vi "PLAN IN UNLOADING SCREEN.vi"(11 "Unloading cyc Data":T1) -> (0 "Unloading cyc Data 2":T1, 1 "Bin/Box":i32, 2 "PLAN DATA Out":string[][](array[string]), 3 "CURRENT PLAN":T2, 5 "FEED CMPLT?":bool)   [LabVIEW 2017]
uses:
  Controls/Unloading_Cyc_Data.ctl
panel:
  # "DOOR NUMBER"
  # "FEEDER STATUS"
  # "DOOR NUMBER"
  # "FEEDER STATUS"
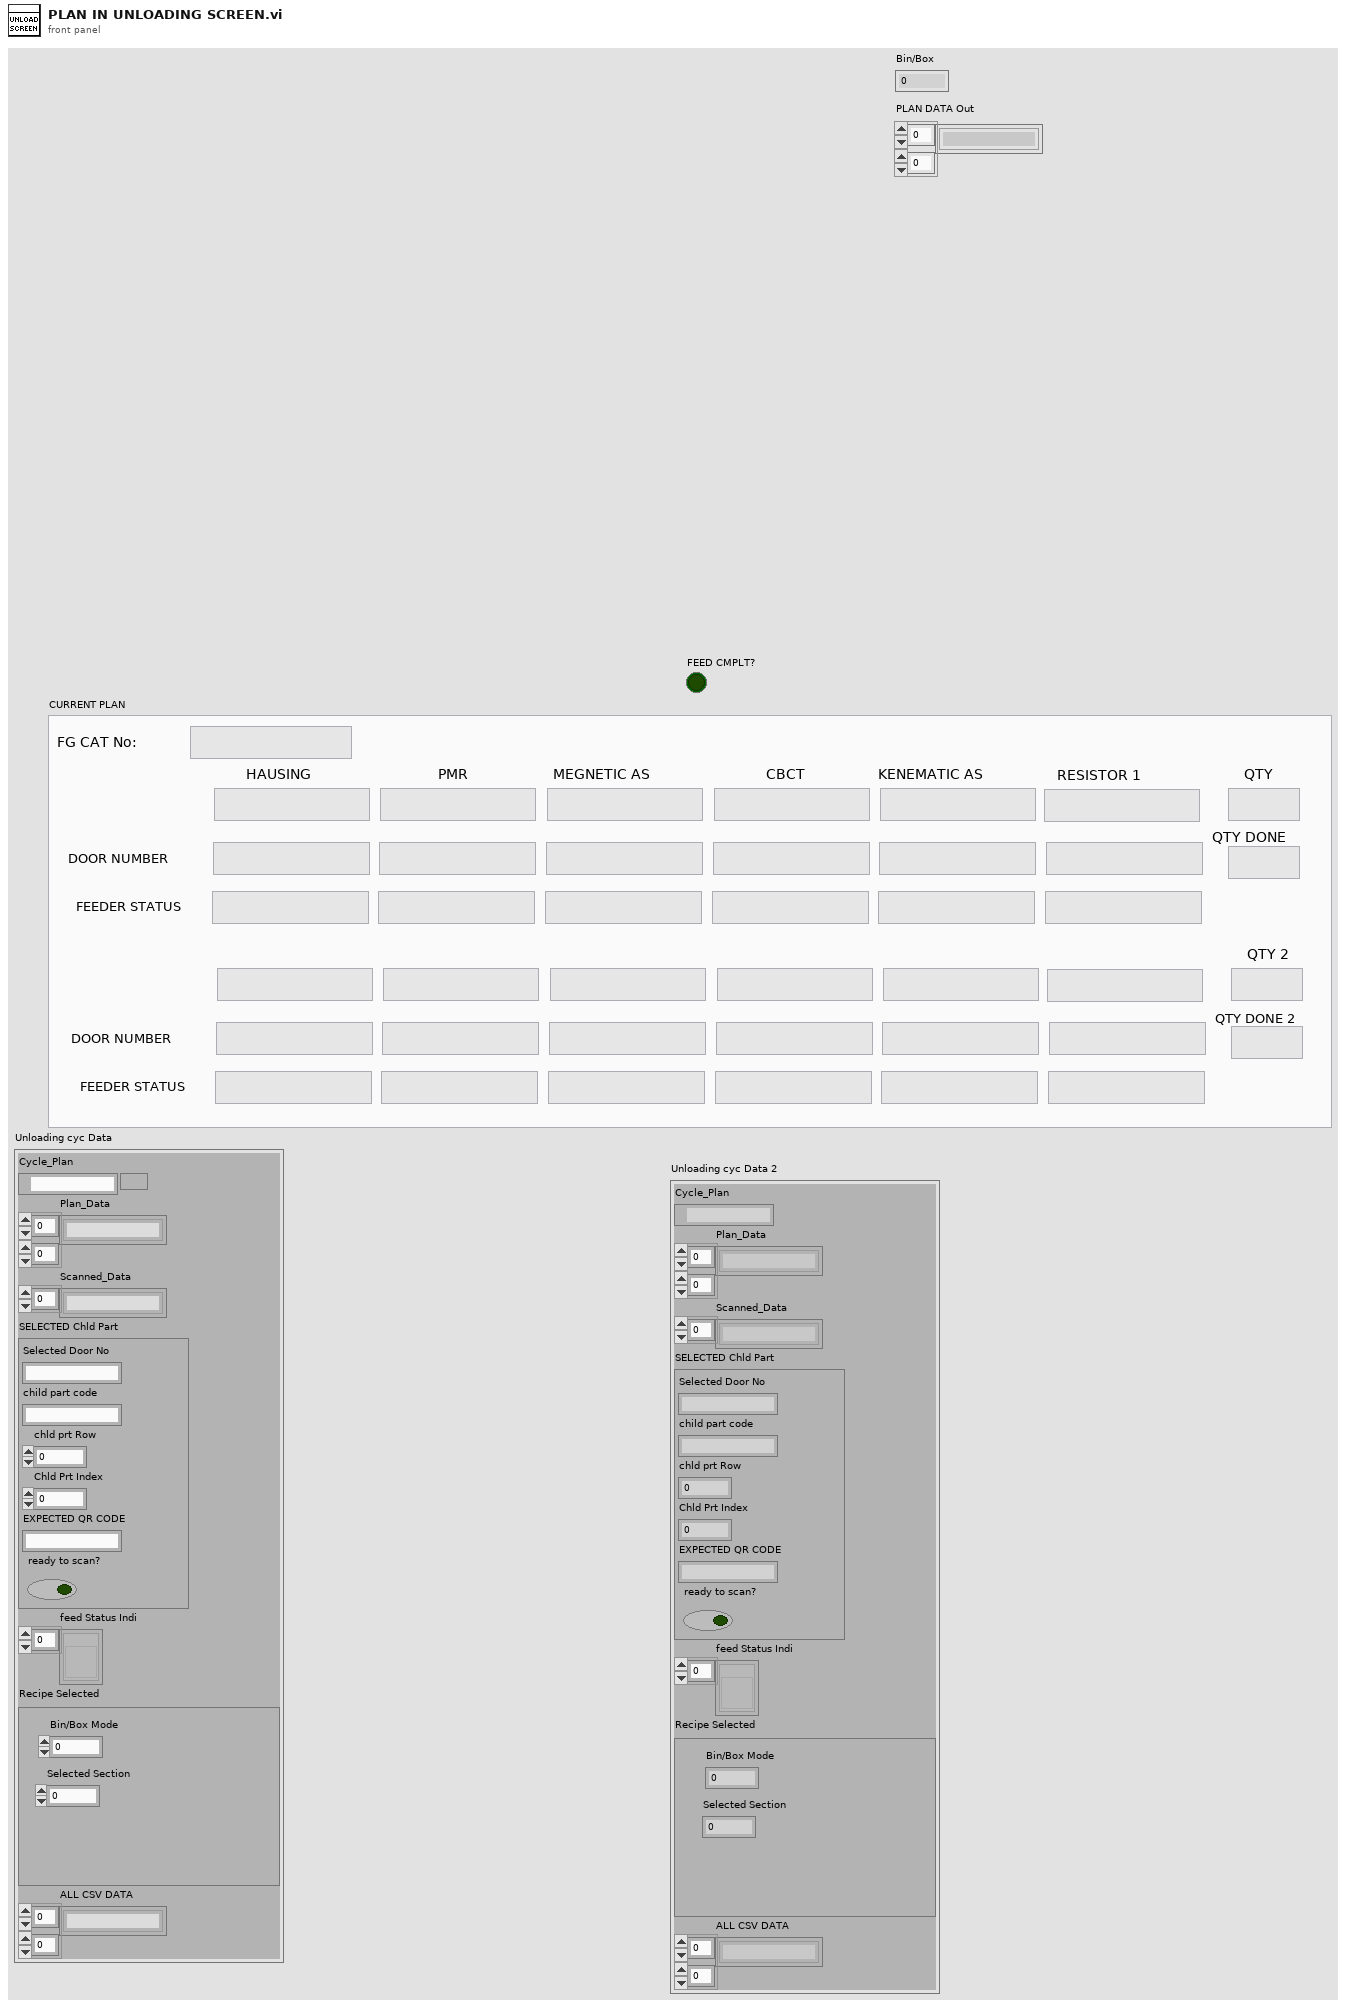
[diagram p1: front panel]
types:
  T1 = typedef "Unloading_Cyc_Data.ctl" = cluster{"Cycle_Plan":path, "Plan_Data":string[][], "Scanned_Data":string[], "SELECTED Chld Part":cluster{"Selected Door No":string, "child part code":string, "chld prt Row":i32, "Chld Prt Index":i32, "EXPECTED QR CODE":string, "ready to scan?":bool}, "feed Status Indi":refnum<vi>[], "Recipe Selected":cluster{"Bin/Box Mode":i32, "Selected Section":i32}, "ALL CSV DATA":string[][]}
  T2 = cluster{"FG CAT No:":string, "HAUSING":string, "PMR":string, "MEGNETIC AS":string, "CBCT":string, "KENEMATIC AS":string, "RESISTOR 1":string, "HAUSING DOOR":string, "PMR DOOR":string, "MAGNETIC AS DOOR":string, "CBCT DOOR":string, "KINEMATIC AS DOOR":string, "RESISTOR 1 DOOR":string, "HAUSING FEED STATUS":string, "PMR FEED STATUS":string, "MAGNETIC AS FEEED STATUS":string, "CBCT FEED STATUS":string, "KINEMATIC AS FEED STATUS":string, "RESISTOR 1 FEED STATUS":string, "QTY":string, "QTY DONE":string, "HAUSING 2":string, "PMR 2":string, "MEGNETIC AS 2":string, "CBCT 2":string, "KENEMATIC AS 2":string, "RESISTOR 2":string, "HAUSING DOOR 2":string, "PMR DOOR 2":string, "MAGNETIC AS DOOR 2":string, "CBCT DOOR 2":string, "KINEMATIC AS DOOR 2":string, "RESISTOR 1 DOOR 2":string, "HAUSING FEED STATUS 2":string, "PMR FEED STATUS 2":string, "MAGNETIC AS FEEED STATUS 2":string, "CBCT FEED STATUS 2":string, "KINEMATIC AS FEED STATUS 2":string, "RESISTOR 1 FEED STATUS 2":string, "QTY 2":string, "QTY DONE 2":string}
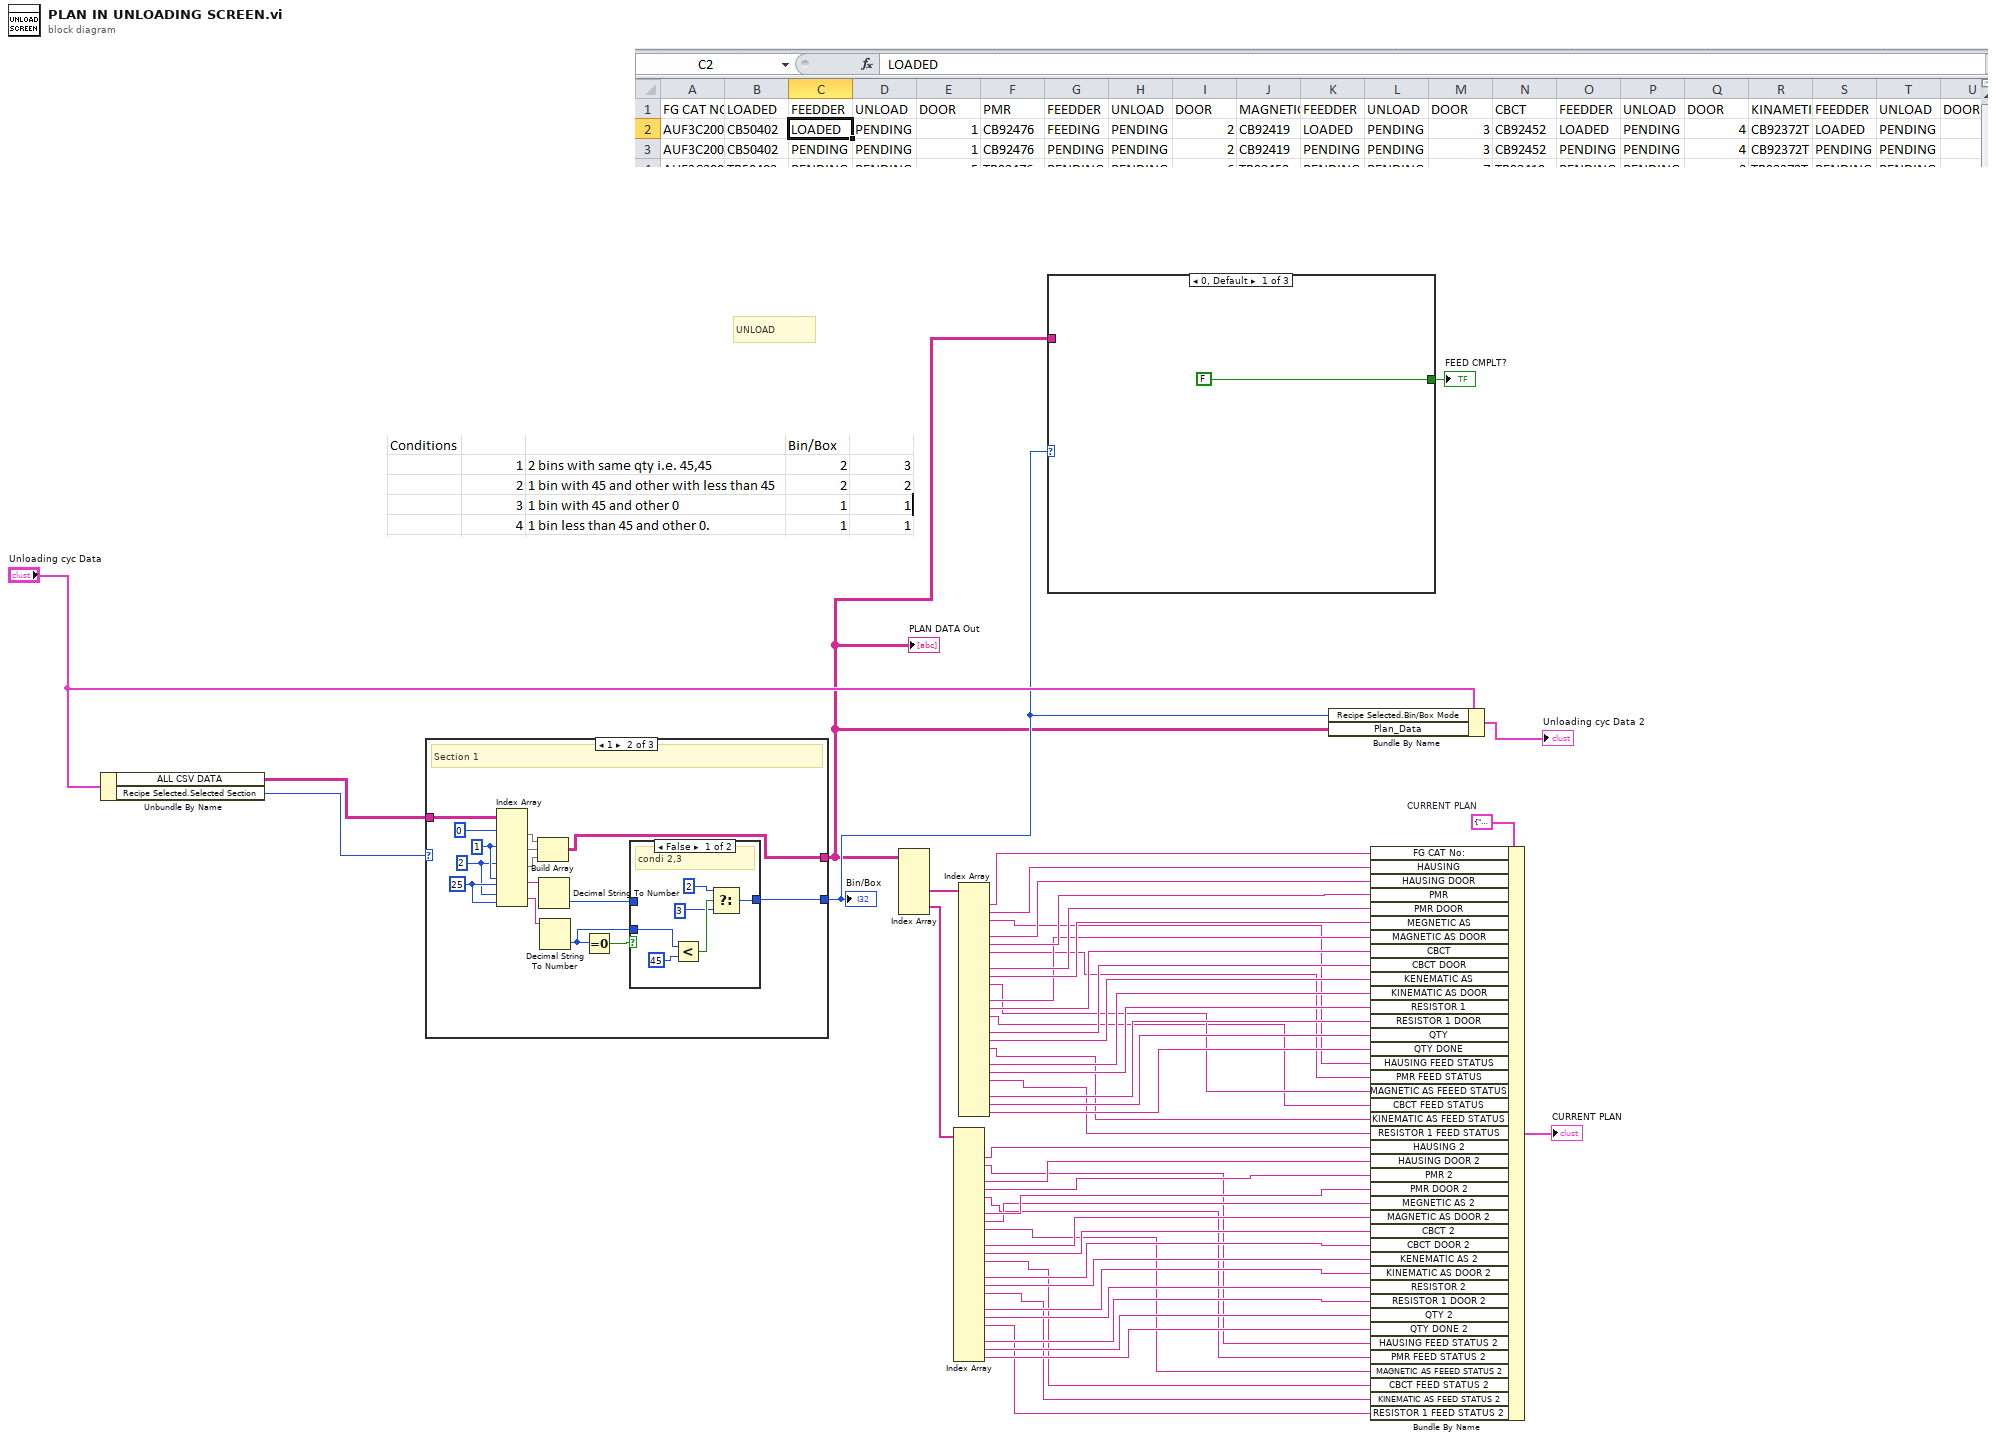
[diagram p0: block diagram]
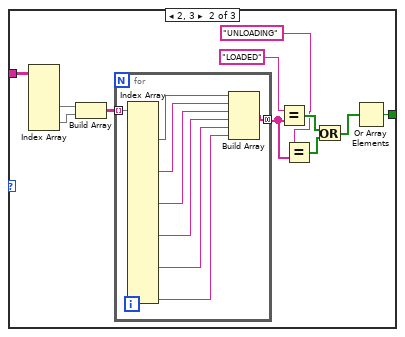
[diagram p2: hidden frame]
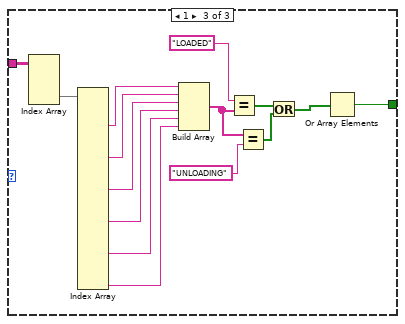
[diagram p3: hidden frame]
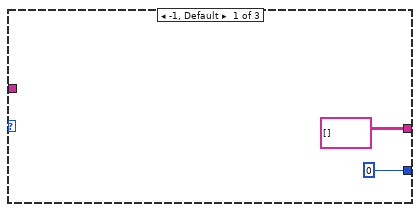
[diagram p4: hidden frame]
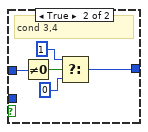
[diagram p5: hidden frame]
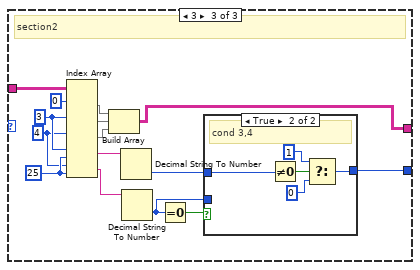
[diagram p6: hidden frame]
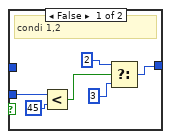
[diagram p7: hidden frame]
diagram:
  w19 = T2 {"FG CAT No:"="", "HAUSING"="", "PMR"="", "MEGNETIC AS"="", "CBCT"="", "KENEMATIC AS"="", "RESISTOR 1"="", "HAUSING DOOR"="", "PMR DOOR"="", "MAGNETIC AS DOOR"="", "CBCT DOOR"="", "KINEMATIC AS DOOR"="", "RESISTOR 1 DOOR"="", "HAUSING FEED STATUS"="", "PMR FEED STATUS"="", "MAGNETIC AS FEEED STATUS"="", "CBCT FEED STATUS"="", "KINEMATIC AS FEED STATUS"="", "RESISTOR 1 FEED STATUS"="", "QTY"="", "QTY DONE"="", "HAUSING 2"="", "PMR 2"="", "MEGNETIC AS 2"="", "CBCT 2"="", "KENEMATIC AS 2"="", "RESISTOR 2"="", "HAUSING DOOR 2"="", "PMR DOOR 2"="", "MAGNETIC AS DOOR 2"="", "CBCT DOOR 2"="", "KINEMATIC AS DOOR 2"="", "RESISTOR 1 DOOR 2"="", "HAUSING FEED STATUS 2"="", "PMR FEED STATUS 2"="", "MAGNETIC AS FEEED STATUS 2"="", "CBCT FEED STATUS 2"="", "KINEMATIC AS FEED STATUS 2"="", "RESISTOR 1 FEED STATUS 2"="", "QTY 2"="", "QTY DONE 2"=""}  # CURRENT PLAN
  # "UNLOAD"
  n1 = Unbundle By Name("Unloading cyc Data") -> ("ALL CSV DATA"=w6:string[][], "Recipe Selected.Selected Section"=w1:i32)
  n2 = case shown="1" w1 {
    tunnel: w6 -> [_ w64 w95]
    tunnel: [string[][] [] w65 w91] -> w2
    tunnel: [0 w56 w89] -> w3
    frame -1, Default {
    }
    frame 1 {
      w62 = 25
      w61 = 2
      w63 = 1
      # "Section 1"
      n3 = Index Array(array=w64, index (row) #1=0, index (row) #2=w63, index (row) #3=w61, index (row) #4=w63, index (col) #4=w62, index (row) #5=w61, index (col) #5=w62) -> (element #1=w67:string[], element #2=w68:string[], element #3=w69:string[], element #4=w59:string, element #5=w60:string)  [unwired: 3 in]
      n4 = Build Array(w67, w68, w69) -> (w65:string[][])
      n5 = Decimal String To Number(string=w59) -> (number=w57:i32)  [unwired: 2 in, 1 out]
      n6 = Decimal String To Number(string=w60) -> (number=w55:i32)  [unwired: 2 in, 1 out]
      n7 = Equal To 0?(x=w55) -> (x = 0?=w58:bool)
      n8 = case shown="False" w58 {
        tunnel: w57 -> [_ w80]
        tunnel: [w73 w76] -> w56
        tunnel: w55 -> [w74 _]
        frame False {
          # "condi 2,3"
          n9 = Less?(x=w74, y=45) -> (x < y?=w71:bool)
          n10 = Select(t=2, s=w71, f=3) -> (s? t:f=w73:i32)
        }
        frame True {
          # "cond 3,4"
          n11 = Not Equal To 0?(x=w80) -> (x != 0?=w79:bool)
          n12 = Select(t=1, s=w79, f=0) -> (s? t:f=w76:i32)
        }
      }
    }
    frame 3 {
      w84 = 25
      w82 = 4
      w83 = 3
      # "section2"
      n13 = Index Array(array=w95, index (row) #1=0, index (row) #2=w83, index (row) #3=w82, index (row) #4=w83, index (col) #4=w84, index (row) #5=w82, index (col) #5=w84) -> (element #1=w94:string[], element #2=w93:string[], element #3=w92:string[], element #4=w86:string, element #5=w85:string)  [unwired: 3 in]
      n14 = Build Array(w94, w93, w92) -> (w91:string[][])
      n15 = Decimal String To Number(string=w86) -> (number=w88:i32)  [unwired: 2 in, 1 out]
      n16 = Decimal String To Number(string=w85) -> (number=w81:i32)  [unwired: 2 in, 1 out]
      n17 = Equal To 0?(x=w81) -> (x = 0?=w87:bool)
      n18 = case shown="True" w87 {
        tunnel: w88 -> [_ w106]
        tunnel: [w97 w102] -> w89
        tunnel: w81 -> [w96 _]
        frame False {
          # "condi 1,2"
          n19 = Less?(x=w96, y=45) -> (x < y?=w101:bool)
          n20 = Select(t=2, s=w101, f=3) -> (s? t:f=w97:i32)
        }
        frame True {
          # "cond 3,4"
          n21 = Not Equal To 0?(x=w106) -> (x != 0?=w105:bool)
          n22 = Select(t=1, s=w105, f=0) -> (s? t:f=w102:i32)
        }
      }
    }
  }
  "PLAN DATA Out" <- w2
  "Bin/Box" <- w3
  n23 = Index Array(array=w2) -> (element #2=w52:string[], element #3=w37:string[])  [unwired: 6 in, 1 out]
  n24 = Index Array(array=w37) -> (element #2=w36:string, element #3=w12:string, element #5=w35:string, element #6=w34:string, element #7=w11:string, element #9=w33:string, element #10=w32:string, element #11=w10:string, element #13=w31:string, element #14=w30:string, element #15=w9:string, element #17=w29:string, element #18=w28:string, element #19=w8:string, element #21=w27:string, element #22=w26:string, element #23=w7:string, element #25=w25:string, element #26=w24:string, element #27=w22:string)  [unwired: 27 in, 7 out]
  n25 = Index Array(array=w52) -> (element #1=w51:string, element #2=w50:string, element #3=w18:string, element #5=w49:string, element #6=w48:string, element #7=w17:string, element #9=w47:string, element #10=w46:string, element #11=w16:string, element #13=w45:string, element #14=w44:string, element #15=w15:string, element #17=w43:string, element #18=w42:string, element #19=w14:string, element #21=w41:string, element #22=w40:string, element #23=w13:string, element #25=w39:string, element #26=w38:string, element #27=w23:string)  [unwired: 27 in, 6 out]
  n26 = case shown="0, Default" w3 {
    tunnel: w2 -> [_ w118 w141]
    tunnel: [FALSE w113 w132] -> w21
    frame 0, Default {
    }
    frame 2, 3 {
      n27 = Index Array(array=w118) -> (element #2=w117:string[], element #3=w116:string[])  [unwired: 6 in, 1 out]
      n28 = Build Array(w117, w116) -> (w115:string[][])
      n29 = for {
        tunnel: w115 -> [w126] mode=indexing
        tunnel: [w119] -> w109 mode=concatenating
        n30 = Index Array(array=w126) -> (element #3=w125:string, element #7=w124:string, element #11=w123:string, element #15=w122:string, element #19=w121:string, element #23=w120:string)  [unwired: 23 in, 17 out]
        n31 = Build Array(w125, w124, w123, w122, w121, w120) -> (w119:string[])
      }
      n32 = Equal?(x="LOADED", y=w109) -> (x = y?=w111:bool[])
      n33 = Equal?(x="UNLOADING", y=w109) -> (x = y?=w112:bool[])
      n34 = Or(x=w111, y=w112) -> (x .or. y?=w110:bool[])
      n35 = Or Array Elements(Boolean array=w110) -> (logical OR=w113:bool)
    }
    frame 1 {
      n36 = Index Array(array=w141) -> (element #2=w140:string[])  [unwired: 4 in, 1 out]
      n37 = Index Array(array=w140) -> (element #3=w138:string, element #7=w137:string, element #11=w136:string, element #15=w135:string, element #19=w134:string, element #23=w133:string)  [unwired: 23 in, 17 out]
      n38 = Build Array(w138, w137, w136, w135, w134, w133) -> (w128:string[])
      n39 = Equal?(x="LOADED", y=w128) -> (x = y?=w131:bool[])
      n40 = Equal?(x=w128, y="UNLOADING") -> (x = y?=w127:bool[])
      n41 = Or(x=w131, y=w127) -> (x .or. y?=w130:bool[])
      n42 = Or Array Elements(Boolean array=w130) -> (logical OR=w132:bool)
    }
  }
  "FEED CMPLT?" <- w21
  n43 = Bundle By Name(cluster="Unloading cyc Data", "Recipe Selected.Bin/Box Mode"=w3, "Plan_Data"=w2) -> (→"Unloading cyc Data 2":T1)
  n44 = Bundle By Name(cluster=w19, "FG CAT No:"=w51, "HAUSING"=w50, "HAUSING DOOR"=w49, "PMR"=w48, "PMR DOOR"=w47, "MEGNETIC AS"=w46, "MAGNETIC AS DOOR"=w45, "CBCT"=w44, "CBCT DOOR"=w43, "KENEMATIC AS"=w42, "KINEMATIC AS DOOR"=w41, "RESISTOR 1"=w40, "RESISTOR 1 DOOR"=w39, "QTY"=w38, "QTY DONE"=w23, "HAUSING FEED STATUS"=w18, "PMR FEED STATUS"=w17, "MAGNETIC AS FEEED STATUS"=w16, "CBCT FEED STATUS"=w15, "KINEMATIC AS FEED STATUS"=w14, "RESISTOR 1 FEED STATUS"=w13, "HAUSING 2"=w36, "HAUSING DOOR 2"=w35, "PMR 2"=w34, "PMR DOOR 2"=w33, "MEGNETIC AS 2"=w32, "MAGNETIC AS DOOR 2"=w31, "CBCT 2"=w30, "CBCT DOOR 2"=w29, "KENEMATIC AS 2"=w28, "KINEMATIC AS DOOR 2"=w27, "RESISTOR 2"=w26, "RESISTOR 1 DOOR 2"=w25, "QTY 2"=w24, "QTY DONE 2"=w22, "HAUSING FEED STATUS 2"=w12, "PMR FEED STATUS 2"=w11, "MAGNETIC AS FEEED STATUS 2"=w10, "CBCT FEED STATUS 2"=w9, "KINEMATIC AS FEED STATUS 2"=w8, "RESISTOR 1 FEED STATUS 2"=w7) -> (→"CURRENT PLAN":T2)
